vi "test udp++.vi"() -> ()   [LabVIEW 2017]
uses:
  <vilib>/Platform/TimedLoop/XDataNode/timing_clust.ctl
  <vilib>/Platform/TimedLoop/XDataNode/nitl_modes.ctl
  <vilib>/Platform/TimedLoop/XDataNode/wakeup.ctl
  16e1070c-7dc9-4f03-9a7c-c4bc31601776.vi
  dd86c118-00dc-4621-9a13-23dbe0247810.vi
  <vilib>/Utility/High Resolution Relative Seconds.vi
  16e1070c-7dc9-4f03-9a7c-c4bc31601776.vi/c01658a1-883f-489e-b376-c551e55a1c83.vi
  dd86c118-00dc-4621-9a13-23dbe0247810.vi/f576cfcf-0274-437d-9d31-e81457e56e77.vi
  SplitUDPPacks.vi
  <userlib>/_OpenG.lib/comparison/comparison.llb/Data Changed__ogtk.vi
  <userlib>/_OpenG.lib/comparison/comparison.llb/I32 Changed__ogtk.vi
  <vilib>/Platform/TimedLoop/XDataNode/XDataNode.xnode
  <vilib>/Platform/TimedLoop/XDataNode/XDNodeRunTimeDep.lvlib
panel:
  in  "stop":bool
  out "sumcheck 2":dbl[](array[numeric])
  out "sumcheck":dbl
  out "# Count":i64[](array[numeric])
  out "time diff(s)":dbl
  in  "Numeric":i32=500
  out "Array":sgl[](array[numeric])
  out "接收控制指令":sgl[](array[numeric])
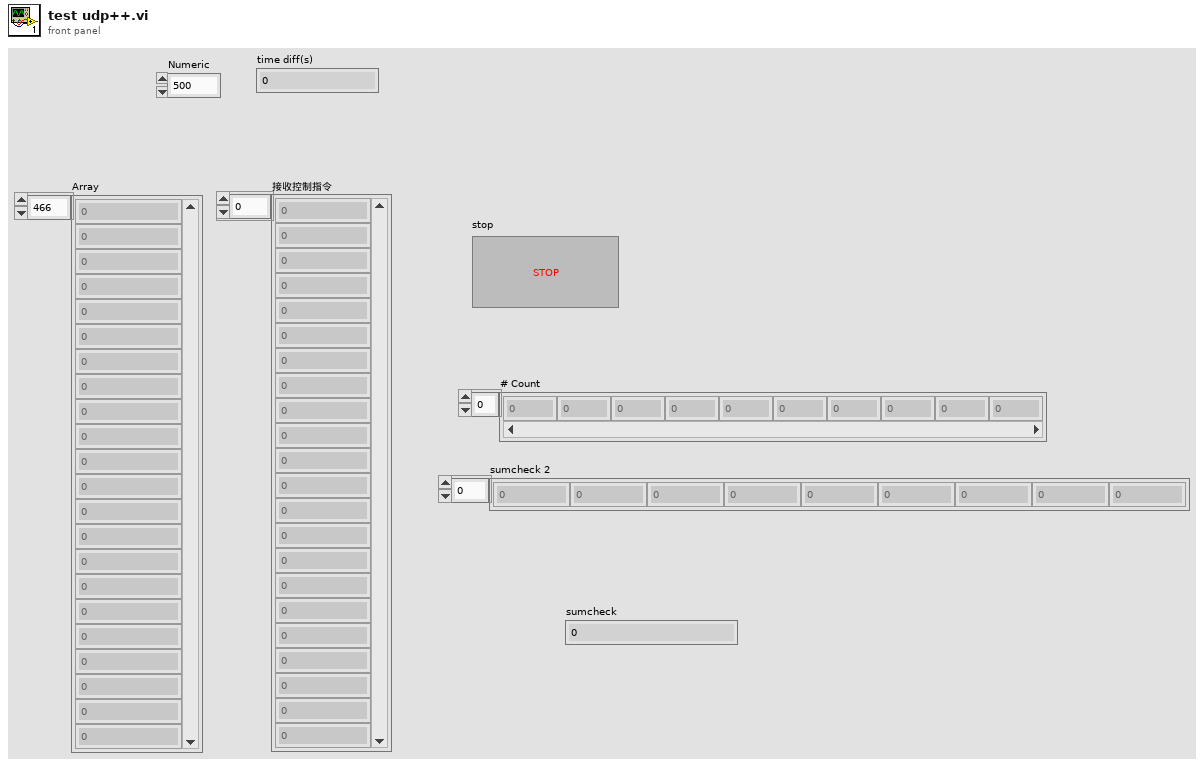
[diagram p1: front panel]
types:
  T1 = cluster{"本地IP":string, "本地端口":u16, "远程IP":string, "远程端口":u16}
  T2 = typedef "XDNodeRunTimeDep.lvlib/timing_clust.ctl" = cluster{"Expected End [f-1]":u64, "Actual End [f-1]":u64, "Finished Late? [f-1]":bool, "Expected End [i-1]":u64, "Actual End [i-1]":u64, "Finished Late? [i-1]":bool, "Expected Start [i]":u64, "Actual Start [i]":u64, "Expected Start [f]":u64, "Actual Start [f]":u64, "Source Name":string, "Structure Name":string, "Period":i64, "Deadline":i64, "Offset":i64, "Start":i64, "Priority":i32, "Timeout":i32, "Mode":T3, "Wakeup Reason":T4, "Error":errorcluster, "Source Type":string, "Secondary Source Type":string, "Global End Time":u64, "Global Start Time":u64, "Frame Duration":u64, "Iteration Duration":u64, "Assigned CPU":i32, "I/O Scan Engine Mode":u32}
  T3 = typedef "XDNodeRunTimeDep.lvlib/nitl_modes.ctl" = enum32{"No Change", "Process missed periods, maintain original phase", "Discard missed periods, maintain original phase", "Process missed periods, ignore original phase", "Discard missed periods, ignore original phase"}
  T4 = typedef "XDNodeRunTimeDep.lvlib/wakeup.ctl" = enum32{"Normal", "Aborted", "Asynchronous wakeup", "Timing source error", "Timed loop error", "Timeout"}
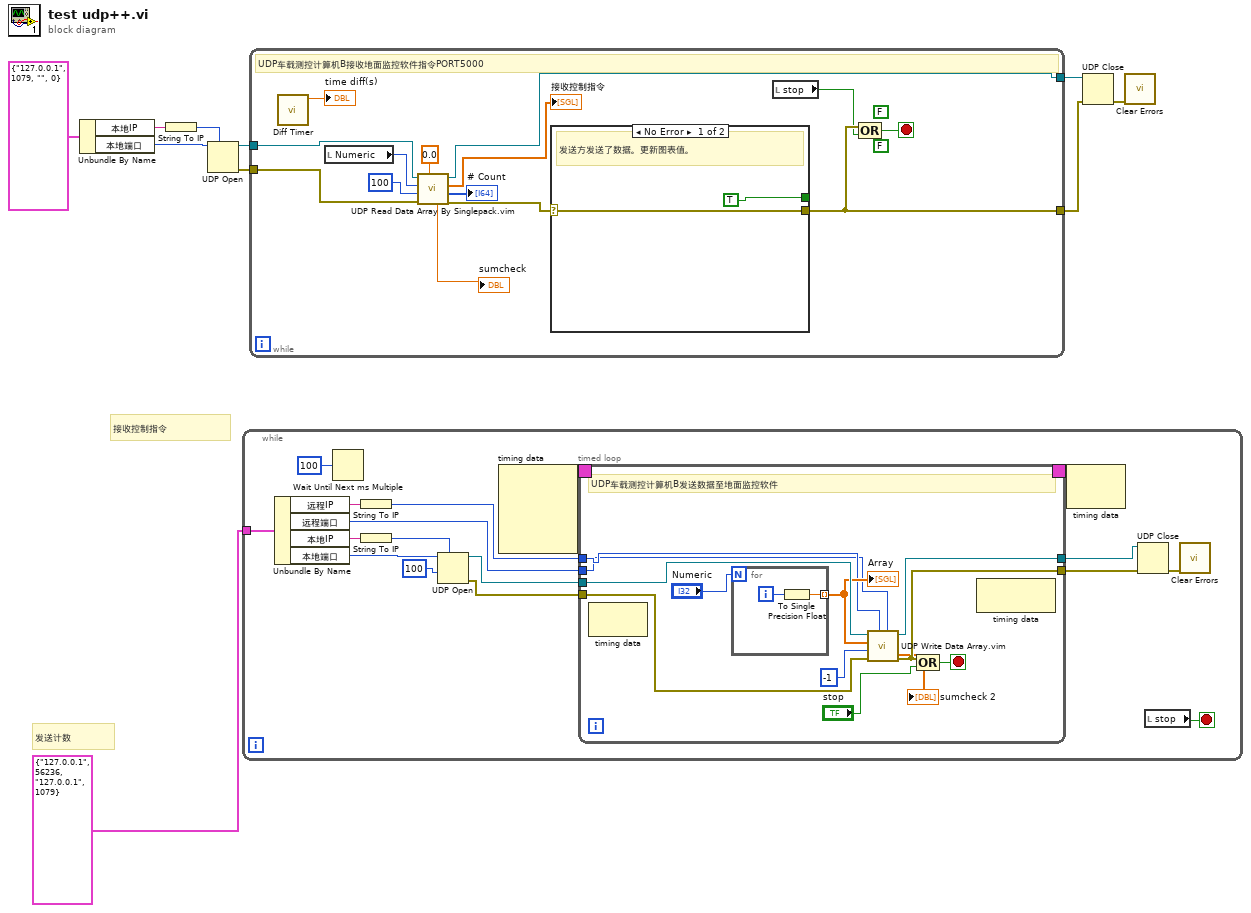
[diagram p0: block diagram]
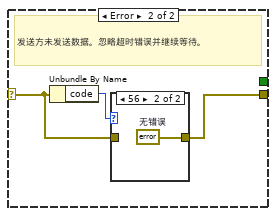
[diagram p2: hidden frame]
diagram:
  # "发送计数"
  # "接收控制指令"
  n1 = Unbundle By Name(T1 {"本地IP"="127.0.0.1", "本地端口"=1079, "远程IP"="", "远程端口"=0} ("UDP配置")) -> ("本地IP"=w3:string, "本地端口"=w2:u16)
  n2 = String To IP(1:w3) -> (0:w10:u32)
  n3 = UDP Open(7:w10, 11:w2) -> (port=w9:refnum<k16>, 0:w8:errorcluster)  [unwired: 3 in, 1 out]
  n4 = while {
    tunnel: T1 {"本地IP"="127.0.0.1", "本地端口"=56236, "远程IP"="127.0.0.1", "远程端口"=1079} ("UDP配置") -> [w16]
    stop <- w11 stop-if-true
    n5 = Unbundle By Name(w16) -> ("远程IP"=w13:string, "远程端口"=w12:u16, "本地IP"=w14:string, "本地端口"=w15:u16)
    n6 = Wait Until Next ms Multiple(millisecond multiple=u32 100 ("毫秒倍数")) -> ()  [unwired: 1 out]
    n7 = String To IP(1:w13) -> (0:w21:u32)
    n8 = String To IP(1:w14) -> (0:w23:u32)
    n9 = UDP Open(7:w23, 9:100 ("超时毫秒(25000)"), 11:w15) -> (port=w25:refnum<k16>, 0:w24:errorcluster)  [unwired: 2 in, 1 out]
    n10 = node-c288() -> (w27:T2)  [unwired: 4 in]
    n11 = timed-loop {
      tunnel: [w36] -> w19
      tunnel: w25 -> [w39]
      tunnel: w24 -> [w37]
      tunnel: [w38] -> w18
      tunnel: w12 -> [w31]
      timing: w27 -> [_]
      timing-out: [_] -> w26
      tunnel: w21 -> [w32]
      stop <- w35 stop-if-true
      # "UDP车载测控计算机B发送数据至地面监控软件"
      n12 = node-c288() -> ()  [unwired: 1 in, 1 out]
      n13 = for {
        N: "Numeric" -> [_]
        tunnel: [w40] -> w33 mode=indexing
        i -> [w41]
        n14 = To Single Precision Float(number=w41) -> (single precision float=w40:sgl)
      }
      "Array" <- w33
      n15 = call "UDP Write Data Array.vim"("port or service name"=w31, "address"=w32, "error in (no error)"=w37, "超时毫秒(25000)"=-1, "Data"=w33, "UDP Network Connection in"=w39) -> ("error out"=w36:errorcluster, "UDP Network Connection out"=w38:refnum<k16>, "checksum"=→"sumcheck 2":dbl[])  [unwired: 3 in]
      n16 = Compound Arithmetic op=OR ("复合运算")(w36, "stop") -> (w35:bool)
      n17 = node-c288() -> ()  [unwired: 1 in, 1 out]
    }
    n18 = node-c288(w26) -> ()  [unwired: 1 out]
    n19 = UDP Close(connection ID=w18, 8:w19) -> (error out=w17:errorcluster)  [unwired: 1 out]
    n20 = local read "stop"() -> (w11:bool)
    n21 = call <vilib>:"Clear Errors.vi"("error in (no error)"=w17) -> ()  [unwired: 5 in, 2 out]
  }
  n22 = while {
    tunnel: w9 -> [w59]
    tunnel: [w57] -> w6
    tunnel: w8 -> [w58]
    tunnel: [w56] -> w7
    stop <- w55 stop-if-true
    (unwired) FALSE ("reset value")
    (unwired) FALSE ("reset")
    # "UDP车载测控计算机B接收地面监控软件指令PORT5000"
    n23 = call "Diff Timer.vi"() -> ("time diff(s)"=→"time diff(s)":dbl)  [unwired: 10 in, 1 out]
    n24 = local read "Numeric"() -> (w51:i32)
    n25 = call "UDP Read Data Array By Singlepack.vim"("Data Type(dbl)"=sgl 0.0, "error in (no error)"=w58, "超时毫秒(25000)"=100 ("timeout ms (25000)"), "total size"=w51, "UDP Network Connection in"=w59) -> ("error out"=w53:errorcluster, "# Count"=→"# Count":i64[], "Array"=→"接收控制指令":sgl[], "UDP Network Connection out"=w57:refnum<k16>, "checksum"=→"sumcheck":dbl)  [unwired: 2 in]
    n26 = case shown="No Error" w53 {
      selector: w53 -> [w61 w63]
      tunnel: [w61 w62] -> w56
      tunnel: [TRUE ("wifi_KongZ") _] -> _
      frame No Error {
        # "发送方发送了数据。更新图表值。"
      }
      frame Error {
        # "发送方未发送数据。忽略超时错误并继续等待。"
        n27 = Unbundle By Name(w63) -> ("code"=w64:i32)
        n28 = case shown="56" w64 {
          tunnel: w63 -> [w65 _]
          tunnel: [w65 w66] -> w62
          frame Default {
          }
          frame 56 {
            w66 = errorcluster {"status"=FALSE, "code"=0, "source"=""}  # 无错误
          }
        }
      }
    }
    n29 = local read "stop"() -> (w46:bool)
    n30 = Compound Arithmetic op=OR ("复合运算")(w56, w46) -> (w55:bool)
  }
  n31 = UDP Close(connection ID=w6, 8:w7) -> (error out=w5:errorcluster)  [unwired: 1 out]
  n32 = call <vilib>:"Clear Errors.vi"("error in (no error)"=w5) -> ()  [unwired: 5 in, 2 out]
